vi "mod_Doppler Interpolating Filter Taps.vi"(0 "interpolation factor":i32=1, 11 "error in (no error)":errorcluster, 13 "reset? (T)":bool=TRUE) -> (4 "interpolating filter taps":dbl[](array[numeric]) format="%.2f", 15 "error out":errorcluster)   [LabVIEW 2020, in "niDMT.lvlib"]
uses:
  <vilib>/addons/Modulation/niDMT.lvlib
  <vilib>/addons/Modulation/niAMT.lvlib
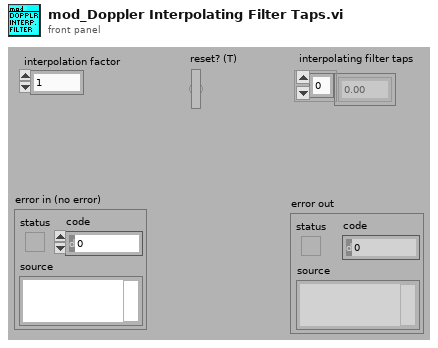
[diagram p1: front panel]
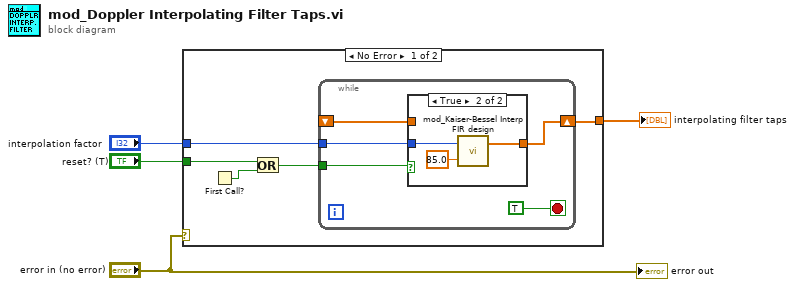
[diagram p0: block diagram]
diagram:
  n1 = case shown="No Error" "error in (no error)" {
    tunnel: "interpolation factor" -> [w7 _]
    tunnel: "reset? (T)" -> [w6 _]
    tunnel: [w5 _] -> w1
    frame No Error {
      n2 = First Call?() -> (First Call?: T/F=w9:bool)
      n3 = Or(x=w6, y=w9) -> (x .or. y?=w8:bool)
      n4 = while {
        shift-right: [w14] -> w5
        shift-left: _ -> [w13]
        tunnel: w8 -> [w11]
        tunnel: w7 -> [w10]
        stop <- TRUE stop-if-true
        n5 = case shown="True" w11 {
          tunnel: [w15 w17] -> w14
          tunnel: w13 -> [w15 _]
          tunnel: w10 -> [_ w16]
          frame False {
          }
          frame True {
            n6 = call <vilib>:"mod_Kaiser-Bessel Interp FIR design.vi"("Stop Attenuation"=85.0, "interpolation factor"=w16) -> ("h"=w17:dbl[])  [unwired: 1 out]
          }
        }
      }
    }
    frame Error {
    }
  }
  "interpolating filter taps" <- w1
  "error out" <- "error in (no error)"
